vi "Brainstorming Canvas.vi"() -> ()   [LabVIEW 2015]
uses:
  <vilib>/Utility/file.llb/Read Delimited Spreadsheet (I64).vi
  <vilib>/Utility/file.llb/Write Delimited Spreadsheet (I64).vi
  Endigit Library/Endigit.lvlib
panel:
  in  "Current Color":u32(colorbox)=16711680
  in  "New Idea":bool
  in  "stop":bool
  in  "Idea":u16(ring) items=["asdf", "Buff line", "Concentri City", "Death Star", "ex", "Expand", "Lattice", "Line Dancer", "Pods", "SVoT"]
  in  "Canvas":u32[][](array[colorbox])
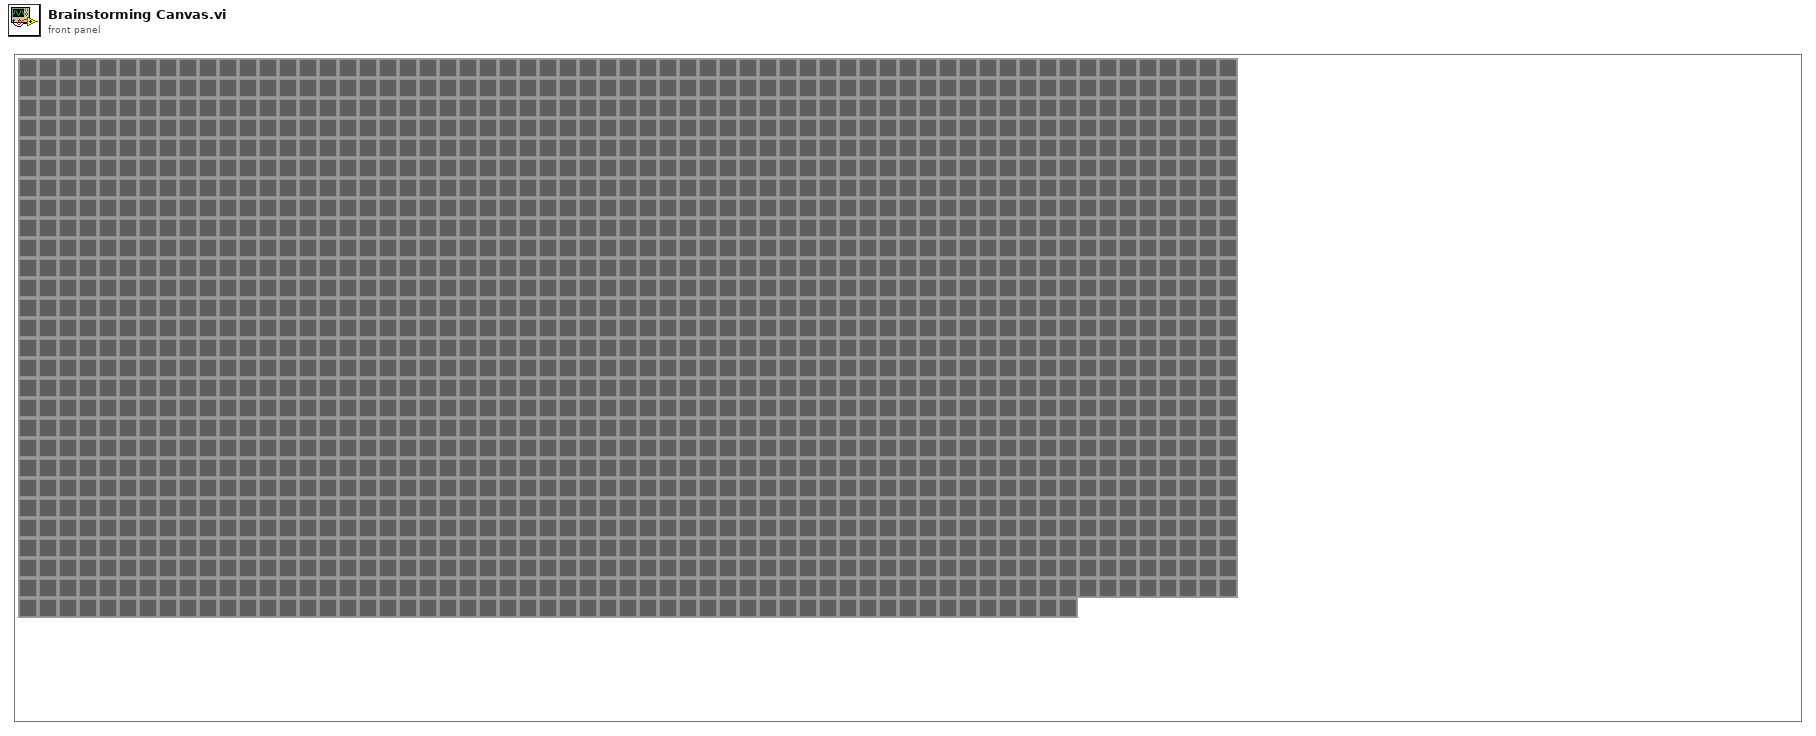
[diagram p1: front panel]
types:
  T1 = typedef "LVPositionTypeDef.ctl" = cluster{"Left":i32, "Top":i32}
  T2 = typedef "LVBoundsTypeDef.ctl" = cluster{"Width":u32, "Height":u32}
  T3 = typedef "LVPoint32TypeDef.ctl" = cluster{"Horizontal":i32, "Vertical":i32}
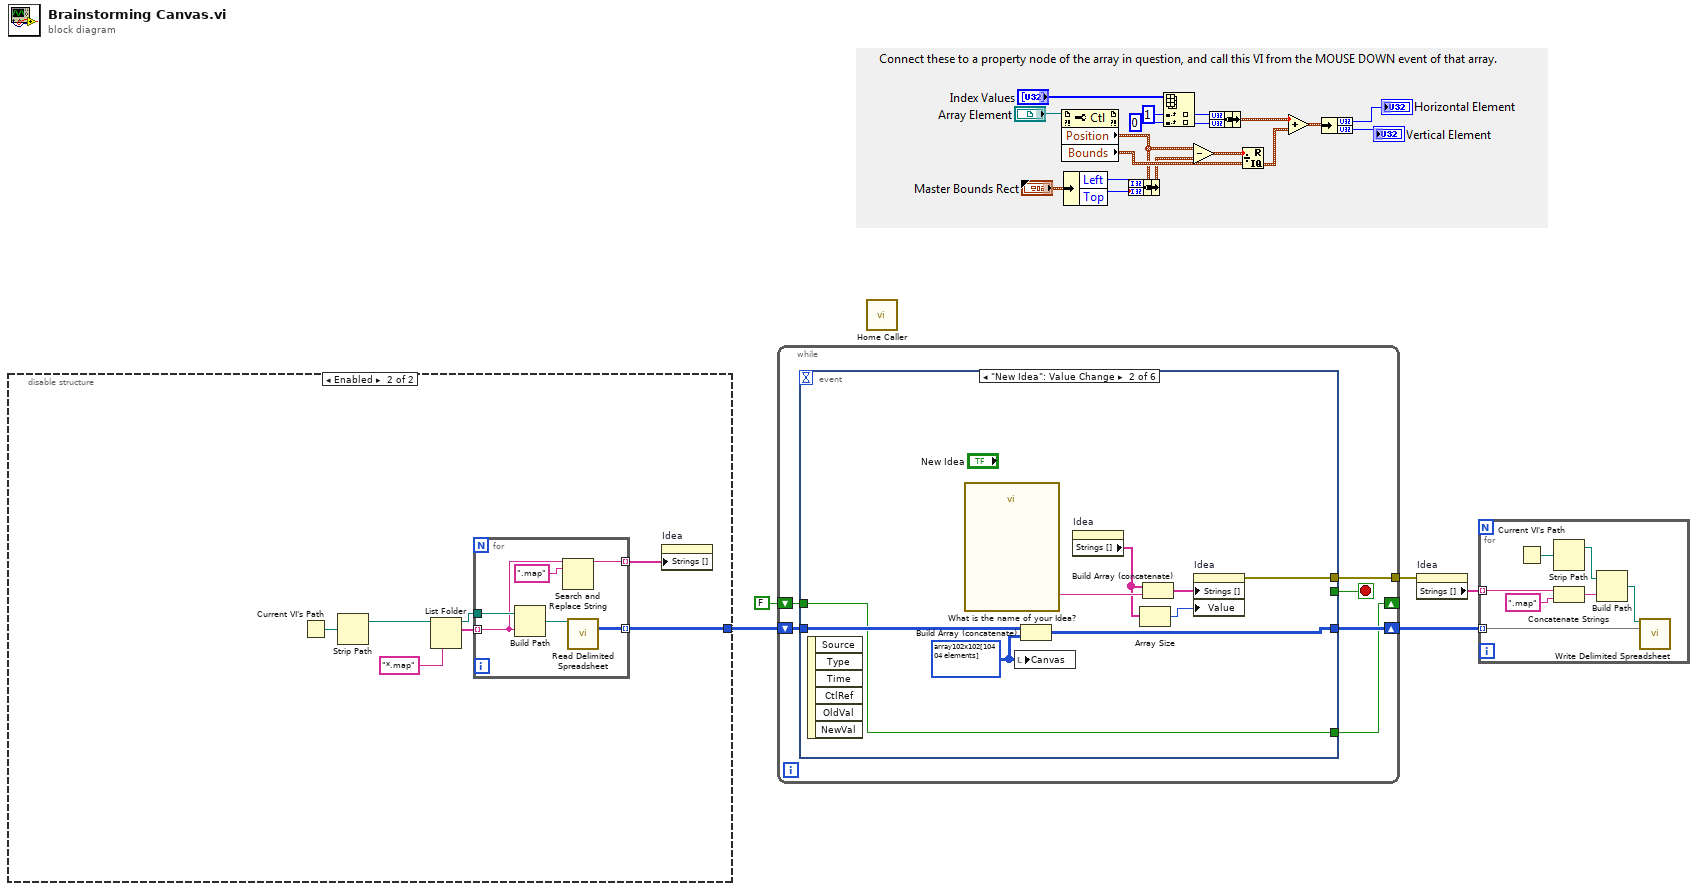
[diagram p0: block diagram]
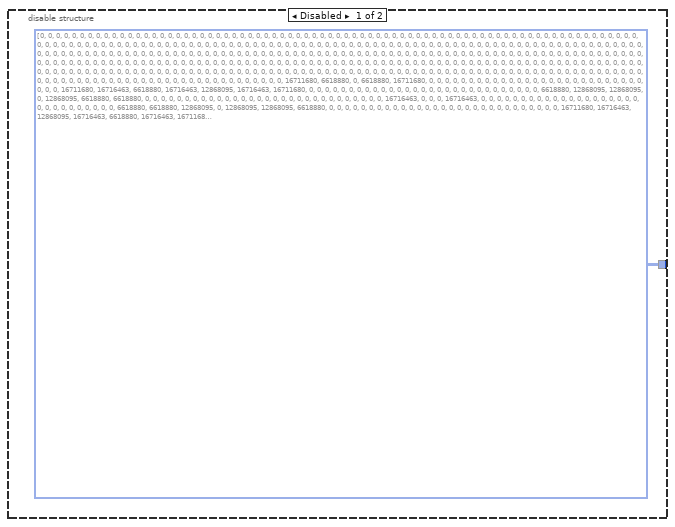
[diagram p2: hidden frame]
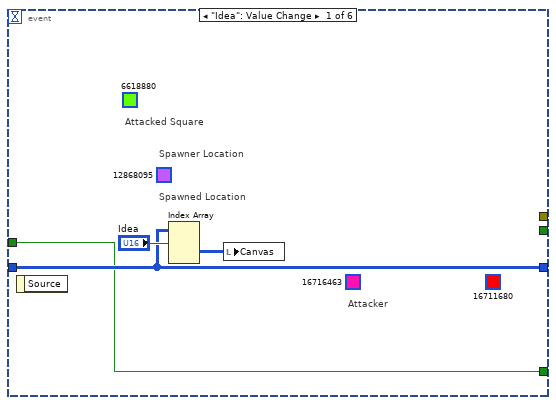
[diagram p3: hidden frame]
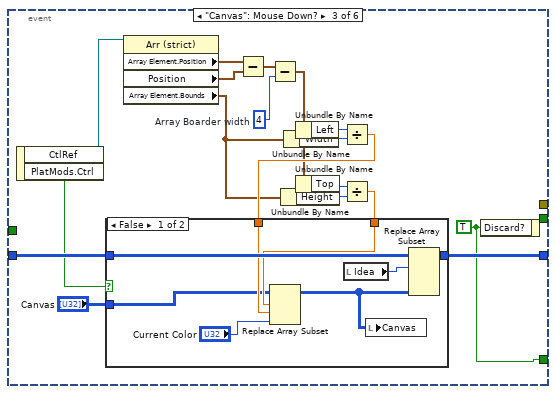
[diagram p4: hidden frame]
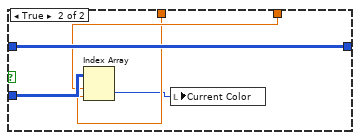
[diagram p5: hidden frame]
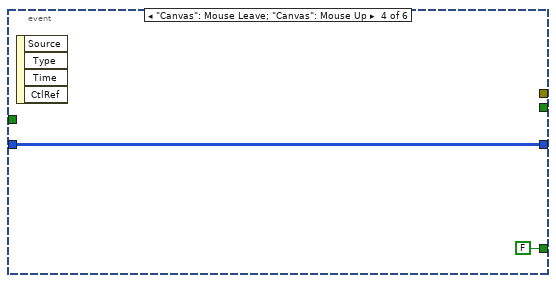
[diagram p6: hidden frame]
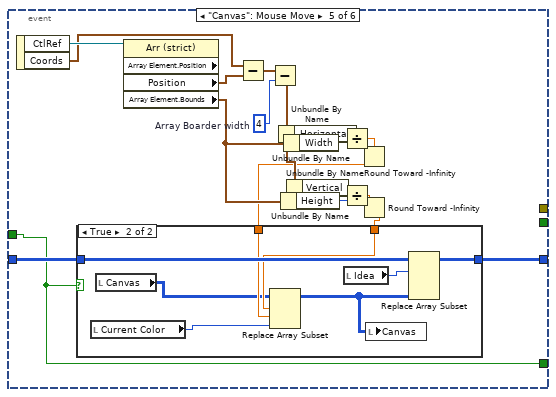
[diagram p7: hidden frame]
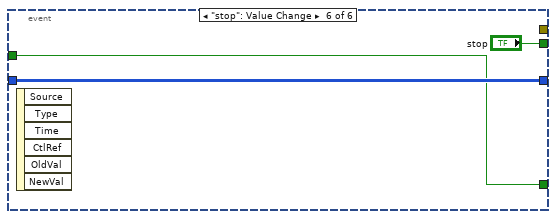
[diagram p9: hidden frame]
diagram:
  n1 = disable-structure shown="Enabled" {
    disable-tunnel: [u32[][][] [[[0, 0, 0, 0, 0, 0, 0, 0, 0, 0, 0, 0, 0, 0, 0, 0, 0, 0, 0, 0, 0, 0, 0, 0, 0, 0, 0, 0, 0, 0, 0, 0, 0, 0, 0, 0], [0, 0, 0, 0, 0, 0, 0, 0, 0, 0, 0, 0, 0, 0, 0, 0, 0, 0, 0, 0, 0, 0, 0, 0, 0, 0, 0, 0, 0, 0, 0, 0, 0, 0, 0, 0], [0, 0, 0, 0, 0, 0, 0, 0, 0, 0, 0, 0, 0, 0, 0, 0, 0, 0, 0, 0, 0, 0, 0, 0, 0, 0, 0, 0, 0, 0, 0, 0, 0, 0, 0, 0], [0, 0, 0, 0, 0, 0, 0, 0, 0, 0, 0, 0, 0, 0, 0, 0, 0, 0, 0, 0, 0, 0, 0, 0, 0, 0, 0, 0, 0, 0, 0, 0, 0, 0, 0, 0], [0, 0, 0, 0, 0, 0, 0, 0, 0, 0, 0, 0, 0, 0, 0, 0, 0, 0, 0, 0, 0, 0, 0, 0, 0, 0, 0, 0, 0, 0, 0, 0, 0, 0, 0, 0], [0, 0, 0, 0, 0, 0, 0, 0, 0, 0, 0, 0, 0, 0, 0, 0, 0, 0, 0, 0, 0, 0, 0, 0, 0, 0, 0, 0, 0, 0, 0, 0, 0, 0, 0, 0], [0, 0, 0, 0, 0, 0, 0, 0, 0, 0, 0, 0, 0, 0, 0, 0, 0, 0, 0, 0, 0, 0, 0, 0, 0, 0, 0, 0, 0, 0, 0, 0, 0, 0, 0, 0], [0, 0, 0, 0, 0, 0, 0, 0, 0, 0, 0, 0, 0, 0, 0, 0, 0, 0, 0, 0, 0, 0, 0, 0, 0, 0, 0, 0, 0, 0, 0, 0, 0, 0, 0, 0], [0, 0, 0, 0, 0, 0, 0, 0, 0, 0, 0, 0, 0, 0, 0, 0, 0, 0, 0, 0, 0, 0, 0, 0, 0, 0, 0, 0, 0, 0, 0, 0, 0, 0, 0, 0], [0, 0, 0, 0, 0, 0, 0, 0, 0, 0, 0, 0, 0, 0, 0, 0, 0, 0, 0, 0, 0, 0, 0, 0, 0, 0, 0, 0, 0, 0, 0, 0, 0, 0, 0, 0], [0, 0, 0, 0, 0, 0, 0, 0, 0, 0, 0, 0, 0, 0, 0, 0, 0, 0, 0, 0, 0, 0, 0, 0, 0, 0, 0, 0, 0, 0, 0, 0, 0, 0, 0, 0], [0, 0, 0, 0, 0, 0, 0, 0, 0, 0, 0, 0, 0, 0, 16711680, 6618880, 0, 6618880, 16711680, 0, 0, 0, 0, 0, 0, 0, 0, 0, 0, 0, 0, 0, 0, 0, 0, 0], [0, 0, 0, 0, 0, 0, 0, 0, 0, 0, 0, 0, 0, 16711680, 16716463, 6618880, 16716463, 12868095, 16716463, 16711680, 0, 0, 0, 0, 0, 0, 0, 0, 0, 0, 0, 0, 0, 0, 0, 0], [0, 0, 0, 0, 0, 0, 0, 0, 0, 0, 0, 0, 0, 6618880, 12868095, 12868095, 0, 12868095, 6618880, 6618880, 0, 0, 0, 0, 0, 0, 0, 0, 0, 0, 0, 0, 0, 0, 0, 0], [0, 0, 0, 0, 0, 0, 0, 0, 0, 0, 0, 0, 0, 0, 16716463, 0, 0, 0, 16716463, 0, 0, 0, 0, 0, 0, 0, 0, 0, 0, 0, 0, 0, 0, 0, 0, 0], [0, 0, 0, 0, 0, 0, 0, 0, 0, 0, 0, 0, 0, 6618880, 6618880, 12868095, 0, 12868095, 12868095, 6618880, 0, 0, 0, 0, 0, 0, 0, 0, 0, 0, 0, 0, 0, 0, 0, 0], [0, 0, 0, 0, 0, 0, 0, 0, 0, 0, 0, 0, 0, 16711680, 16716463, 12868095, 16716463, 6618880, 16716463, 16711680, 0, 0, 0, 0, 0, 0, 0, 0, 0, 0, 0, 0, 0, 0, 0, 0], [0, 0, 0, 0, 0, 0, 0, 0, 0, 0, 0, 0, 0, 0, 16711680, 6618880, 0, 6618880, 16711680, 0, 0, 0, 0, 0, 0, 0, 0, 0, 0, 0, 0, 0, 0, 0, 0, 0], [0, 0, 0, 0, 0, 0, 0, 0, 0, 0, 0, 0, 0, 0, 0, 0, 0, 0, 0, 0, 0, 0, 0, 0, 0, 0, 0, 0, 0, 0, 0, 0, 0, 0, 0, 0], [0, 0, 0, 0, 0, 0, 0, 0, 0, 0, 0, 0, 0, 0, 0, 0, 0, 0, 0, 0, 0, 0, 0, 0, 0, 0, 0, 0, 0, 0, 0, 0, 0, 0, 0, 0], [0, 0, 0, 0, 0, 0, 0, 0, 0, 0, 0, 0, 0, 0, 0, 0, 0, 0, 0, 0, 0, 0, 0, 0, 0, 0, 0, 0, 0, 0, 0, 0, 0, 0, 0, 0], [0, 0, 0, 0, 0, 0, 0, 0, 0, 0, 0, 0, 0, 0, 0, 0, 0, 0, 0, 0, 0, 0, 0, 0, 0, 0, 0, 0, 0, 0, 0, 0, 0, 0, 0, 0], [0, 0, 0, 0, 0, 0, 0, 0, 0, 0, 0, 0, 0, 0, 0, 0, 0, 0, 0, 0, 0, 0, 0, 0, 0, 0, 0, 0, 0, 0, 0, 0, 0, 0, 0, 0], [0, 0, 0, 0, 0, 0, 0, 0, 0, 0, 0, 0, 0, 0, 0, 0, 0, 0, 0, 0, 0, 0, 0, 0, 0, 0, 0, 0, 0, 0, 0, 0, 0, 0, 0, 0], [0, 0, 0, 0, 0, 0, 0, 0, 0, 0, 0, 0, 0, 0, 0, 0, 0, 0, 0, 0, 0, 0, 0, 0, 0, 0, 0, 0, 0, 0, 0, 0, 0, 0, 0, 0], [0, 0, 0, 0, 0, 0, 0, 0, 0, 0, 0, 0, 0, 0, 0, 0, 0, 0, 0, 0, 0, 0, 0, 0, 0, 0, 0, 0, 0, 0, 0, 0, 0, 0, 0, 0], [0, 0, 0, 0, 0, 0, 0, 0, 0, 0, 0, 0, 0, 0, 0, 0, 0, 0, 0, 0, 0, 0, 0, 0, 0, 0, 0, 0, 0, 0, 0, 0, 0, 0, 0, 0], [0, 0, 0, 0, 0, 0, 0, 0, 0, 0, 0, 0, 0, 0, 0, 0, 0, 0, 0, 0, 0, 0, 0, 0, 0, 0, 0, 0, 0, 0, 0, 0, 0, 0, 0, 0], [0, 0, 0, 0, 0, 0, 0, 0, 0, 0, 0, 0, 0, 0, 0, 0, 0, 0, 0, 0, 0, 0, 0, 0, 0, 0, 0, 0, 0, 0, 0, 0, 0, 0, 0, 0]], [[0, 0, 0, 0, 0, 0, 0, 0, 0, 0, 0, 0, 0, 0, 0, 0, 0, 0, 0, 0, 0, 0, 0, 0, 0, 0, 0, 0, 0, 0, 0, 0, 0, 0, 0, 0], [0, 0, 0, 0, 0, 0, 0, 0, 0, 0, 0, 0, 0, 0, 0, 0, 0, 0, 0, 0, 0, 0, 0, 0, 0, 0, 0, 0, 0, 0, 0, 0, 0, 0, 0, 0], [0, 0, 0, 0, 0, 0, 0, 0, 0, 0, 0, 0, 0, 0, 0, 0, 0, 0, 0, 0, 0, 0, 0, 0, 0, 0, 0, 0, 0, 0, 0, 0, 0, 0, 0, 0], [0, 0, 0, 0, 0, 0, 0, 0, 0, 0, 0, 0, 0, 0, 0, 0, 0, 0, 0, 0, 0, 0, 0, 0, 0, 0, 0, 0, 0, 0, 0, 0, 0, 0, 0, 0], [0, 0, 0, 0, 0, 0, 0, 0, 0, 0, 0, 0, 0, 0, 0, 0, 0, 0, 0, 0, 0, 0, 0, 0, 0, 0, 0, 0, 0, 0, 0, 0, 0, 0, 0, 0], [0, 0, 0, 0, 0, 0, 0, 0, 0, 0, 0, 0, 0, 0, 0, 0, 0, 0, 0, 0, 0, 0, 0, 0, 0, 0, 0, 0, 0, 0, 0, 0, 0, 0, 0, 0], [0, 0, 0, 0, 0, 0, 0, 0, 0, 0, 0, 0, 0, 0, 0, 0, 0, 0, 0, 0, 0, 0, 0, 0, 0, 0, 0, 0, 0, 0, 0, 0, 0, 0, 0, 0], [0, 0, 0, 0, 16711680, 16711680, 16711680, 16711680, 16711680, 16711680, 16711680, 16711680, 16711680, 16711680, 0, 0, 0, 0, 0, 0, 0, 0, 0, 0, 0, 0, 0, 0, 0, 0, 0, 0, 0, 0, 0, 0], [0, 0, 16716463, 12868095, 6618880, 6618880, 6618880, 6618880, 6618880, 6618880, 6618880, 6618880, 6618880, 6618880, 12868095, 16716463, 0, 0, 0, 0, 0, 0, 0, 0, 0, 0, 0, 0, 0, 0, 0, 0, 0, 0, 0, 0], [0, 0, 16716463, 12868095, 6618880, 6618880, 6618880, 6618880, 6618880, 6618880, 6618880, 6618880, 6618880, 6618880, 12868095, 16716463, 0, 0, 0, 0, 0, 0, 0, 0, 0, 0, 0, 0, 0, 0, 0, 0, 0, 0, 0, 0], [0, 0, 0, 0, 16711680, 16711680, 16711680, 16711680, 16711680, 16711680, 16711680, 16711680, 16711680, 16711680, 0, 0, 0, 0, 0, 0, 0, 0, 0, 0, 0, 0, 0, 0, 0, 0, 0, 0, 0, 0, 0, 0], [0, 0, 0, 0, 0, 0, 0, 0, 0, 0, 0, 0, 0, 0, 0, 0, 0, 0, 0, 0, 0, 0, 0, 0, 0, 0, 0, 0, 0, 0, 0, 0, 0, 0, 0, 0], [0, 0, 0, 0, 0, 0, 0, 0, 0, 0, 0, 0, 0, 0, 0, 0, 0, 0, 0, 0, 0, 0, 0, 0, 0, 0, 0, 0, 0, 0, 0, 0, 0, 0, 0, 0], [0, 0, 0, 0, 0, 0, 0, 0, 0, 0, 0, 0, 0, 0, 0, 0, 0, 0, 0, 0, 0, 0, 0, 0, 0, 0, 0, 0, 0, 0, 0, 0, 0, 0, 0, 0], [0, 0, 0, 0, 0, 0, 0, 0, 0, 0, 0, 0, 0, 0, 0, 0, 0, 0, 0, 0, 0, 0, 0, 0, 0, 0, 0, 0, 0, 0, 0, 0, 0, 0, 0, 0], [0, 0, 0, 0, 0, 0, 0, 0, 0, 0, 0, 0, 0, 0, 0, 0, 0, 0, 0, 0, 0, 0, 0, 0, 0, 0, 0, 0, 0, 0, 0, 0, 0, 0, 0, 0], [0, 0, 0, 0, 0, 0, 0, 0, 0, 0, 0, 0, 0, 0, 0, 0, 0, 0, 0, 0, 0, 0, 0, 0, 0, 0, 0, 0, 0, 0, 0, 0, 0, 0, 0, 0], [0, 0, 0, 0, 0, 0, 0, 0, 0, 0, 0, 0, 0, 0, 0, 0, 0, 0, 0, 0, 0, 0, 0, 0, 0, 0, 0, 0, 0, 0, 0, 0, 0, 0, 0, 0], [0, 0, 0, 0, 0, 0, 0, 0, 0, 0, 0, 0, 0, 0, 0, 0, 0, 0, 0, 0, 0, 0, 0, 0, 0, 0, 0, 0, 0, 0, 0, 0, 0, 0, 0, 0], [0, 0, 0, 0, 0, 0, 0, 0, 0, 0, 0, 0, 0, 0, 0, 0, 0, 0, 0, 0, 0, 0, 0, 0, 0, 0, 0, 0, 0, 0, 0, 0, 0, 0, 0, 0], [0, 0, 0, 0, 0, 0, 0, 0, 0, 0, 0, 0, 0, 0, 0, 0, 0, 0, 0, 0, 0, 0, 0, 0, 0, 0, 0, 0, 0, 0, 0, 0, 0, 0, 0, 0], [0, 0, 0, 0, 0, 0, 0, 0, 0, 0, 0, 0, 0, 0, 0, 0, 0, 0, 0, 0, 0, 0, 0, 0, 0, 0, 0, 0, 0, 0, 0, 0, 0, 0, 0, 0], [0, 0, 0, 0, 0, 0, 0, 0, 0, 0, 0, 0, 0, 0, 0, 0, 0, 0, 0, 0, 0, 0, 0, 0, 0, 0, 0, 0, 0, 0, 0, 0, 0, 0, 0, 0], [0, 0, 0, 0, 0, 0, 0, 0, 0, 0, 0, 0, 0, 0, 0, 0, 0, 0, 0, 0, 0, 0, 0, 0, 0, 0, 0, 0, 0, 0, 0, 0, 0, 0, 0, 0], [0, 0, 0, 0, 0, 0, 0, 0, 0, 0, 0, 0, 0, 0, 0, 0, 0, 0, 0, 0, 0, 0, 0, 0, 0, 0, 0, 0, 0, 0, 0, 0, 0, 0, 0, 0], [0, 0, 0, 0, 0, 0, 0, 0, 0, 0, 0, 0, 0, 0, 0, 0, 0, 0, 0, 0, 0, 0, 0, 0, 0, 0, 0, 0, 0, 0, 0, 0, 0, 0, 0, 0], [0, 0, 0, 0, 0, 0, 0, 0, 0, 0, 0, 0, 0, 0, 0, 0, 0, 0, 0, 0, 0, 0, 0, 0, 0, 0, 0, 0, 0, 0, 0, 0, 0, 0, 0, 0], [0, 0, 0, 0, 0, 0, 0, 0, 0, 0, 0, 0, 0, 0, 0, 0, 0, 0, 0, 0, 0, 0, 0, 0, 0, 0, 0, 0, 0, 0, 0, 0, 0, 0, 0, 0], [0, 0, 0, 0, 0, 0, 0, 0, 0, 0, 0, 0, 0, 0, 0, 0, 0, 0, 0, 0, 0, 0, 0, 0, 0, 0, 0, 0, 0, 0, 0, 0, 0, 0, 0, 0]]] ("Death Star") w8] -> w2
    frame Disabled {
    }
    frame Enabled {
      n2 = Current VI's Path() -> (path=w10:path)
      n3 = Strip Path(path=w10) -> (stripped path=w7:path)  [unwired: 1 out]
      n4 = List Folder(path=w7, pattern="*.map") -> (path out=w11:path, filenames=w12:string[])  [unwired: 2 in, 2 out]
      n5 = for {
        tunnel: w11 -> [w19]
        tunnel: w12 -> [w15] mode=indexing
        tunnel: [w17] -> w8 mode=indexing
        tunnel: [w14] -> w13 mode=indexing
        n6 = Build Path(base path=w19, name or relative path=w15) -> (appended path=w18:path)
        n7 = Search and Replace String(input string=w15, search string=".map") -> (result string=w14:string)  [unwired: 6 in, 3 out]
        n8 = call-poly <vilib>:"Read Delimited Spreadsheet.vi"("file path (dialog if empty)"=w18) -> ("all rows"=w17:i64[][])  [unwired: 9 in, 5 out]
      }
      n9 = property on="Idea" class="Ring (strict)"("Strings []"=w13) -> ()  [unwired: 2 in, 2 out]
    }
  }
  n10 = while {
    shift-right: [w23] -> w4
    shift-left: w2 -> [w24]
    tunnel: [w22] -> w5
    shift-right: [w20] -> _
    shift-left: FALSE -> [w21]
    stop <- w25 stop-if-true
    n11 = event shown="[1] \"New Idea\": Value Change" {
      selector: _ -> [_ _ _ _ _ _]
      dyn-events: _ -> [_ _ _ _ _ _]
      timeout: _ -> [_ _ _ _ _ _]
      tunnel: [_ _ _ _ _ "stop"] -> w25
      tunnel: w24 -> [w27 w38 w56 w71 w89 w100]
      tunnel: [w27 w35 w55 w71 w88 w100] -> w23
      tunnel: [_ w33 _ _ _ _] -> w22
      tunnel: w21 -> [w26 w32 _ _ w72 w99]
      tunnel: [w26 w32 w39 FALSE ("Discard?") w72 w99] -> w20
      event "Idea": Value Change {
        (unwired) u32 16711680 ("Color Box 17")
        (unwired) u32 6618880 ("Color Box 14")
        (unwired) u32 16716463 ("Color Box 11")
        (unwired) u32 12868095 ("Color Box 12")
        # "Attacked Square"
        # "Attacker"
        # "Spawned Location"
        # "Spawner Location"
        n12 = event-data() -> ()  [unwired: 1 in, 1 out]
        n13 = Index Array(array=w27, index (dim 0)="Idea") -> (element=w28:i64[][])  [unwired: 2 in]
        n14 = local write "Canvas"(w28) -> ()
      }
      event "New Idea": Value Change {
        w34 = u32[][] array102x102[10404 elements] ("Death Star")
        n15 = event-data() -> ()  [unwired: 1 in, 6 out]
        n16 = call "What is the name of your Idea?"() -> ("Idea Name"=w37:string)  [unwired: 17 in, 2 out]
        n17 = local write "Canvas"(w34) -> ()
        n18 = Build Array (concatenate)(w38, w34) -> (w35:i64[][][])
        n19 = property on="Idea" class="Ring (strict)"() -> ("Strings []"=w31:string[])  [unwired: 2 in, 2 out]
        n20 = Array Size(array=w31) -> (size(s)=w30:i32)
        n21 = Build Array (concatenate)(w31, w37) -> (w36:string[])
        n22 = property on="Idea" class="Ring (strict)"("Strings []"=w36, "Value"=w30) -> (error out=w33:errorcluster)  [unwired: 2 in, 1 out]
      }
      event "Canvas": Mouse Down? {
        w51 = 4  # Array Boarder width
        w39 = TRUE ("Discard?")
        n23 = event-data() -> ("CtlRef"=w54:refnum<vi>, "PlatMods.Ctrl"=w41:bool)  [unwired: 1 in]
        n24 = property class="Arr (strict)"(reference=w54) -> ("Array Element.Position"=w42:T1, "Position"=w53:T1, "Array Element.Bounds"=w46:T2)  [unwired: 1 in, 2 out]
        n25 = Subtract(x=w42, y=w53) -> (x-y=w52:T1)
        n26 = Subtract(x=w52, y=w51) -> (x-y=w47:T1)
        n27 = Unbundle By Name(w46) -> ("Height"=w44:u32)
        n28 = Unbundle By Name(w46) -> ("Width"=w49:u32)
        n29 = Unbundle By Name(w47) -> ("Left"=w50:i32)
        n30 = Unbundle By Name(w47) -> ("Top"=w45:i32)
        n31 = Divide(x=w50, y=w49) -> (x/y=w48:dbl)
        n32 = Divide(x=w45, y=w44) -> (x/y=w43:dbl)
        n33 = case shown="False" w41 {
          tunnel: w56 -> [w64 w69]
          tunnel: [w63 w69] -> w55
          tunnel: w48 -> [w60 w66]
          tunnel: w43 -> [w59 w67]
          tunnel: "Canvas" -> [w57 w68]
          frame False {
            n34 = Replace Array Subset(array=w57, new element="Current Color", index (row)=w59, index (col)=w60) -> (w58:u32[][])
            n35 = local read "Idea"() -> (w62:u16)
            n36 = local write "Canvas"(w58) -> ()
            n37 = Replace Array Subset(array=w64, new element=w58, index (dim 0)=w62) -> (w63:i64[][][])  [unwired: 2 in]
          }
          frame True {
            n38 = Index Array(array=w68, index (row)=w67, index (col)=w66) -> (element=w65:u32)
            n39 = local write "Current Color"(w65) -> ()
          }
        }
        n40 = event-data("Discard?"=w39) -> ()  [unwired: 1 in, 1 out]
      }
      event "Canvas": Mouse Leave; "Canvas": Mouse Up {
        n41 = event-data() -> ()  [unwired: 1 in, 4 out]
      }
      event "Canvas": Mouse Move {
        w85 = 4  # Array Boarder width
        n42 = event-data() -> ("CtlRef"=w87:refnum<vi>, "Coords"=w75:T3)  [unwired: 1 in]
        n43 = property class="Arr (strict)" props=["Array Element", "Position", "Position", "Array Element", "Bounds"](reference=w87) -> ("Position"=w76:T1, "Array Element.Bounds"=w80:T2)  [unwired: 1 in, 3 out]
        n44 = Subtract(x=w75, y=w76) -> (x-y=w86:T3)
        n45 = Subtract(x=w86, y=w85) -> (x-y=w81:T3)
        n46 = Unbundle By Name(w81) -> ("Horizontal"=w84:i32)
        n47 = Unbundle By Name(w80) -> ("Height"=w78:u32)
        n48 = Unbundle By Name(w80) -> ("Width"=w83:u32)
        n49 = Unbundle By Name(w81) -> ("Vertical"=w79:i32)
        n50 = Divide(x=w84, y=w83) -> (x/y=w82:dbl)
        n51 = Divide(x=w79, y=w78) -> (x/y=w77:dbl)
        n52 = Round Toward -Infinity(1:w82) -> (0:w73:dbl)
        n53 = Round Toward -Infinity(1:w77) -> (0:w74:dbl)
        n54 = case shown="True" w72 {
          tunnel: w89 -> [w90 w98]
          tunnel: [w90 w97] -> w88
          tunnel: w73 -> [_ w96]
          tunnel: w74 -> [_ w95]
          frame False {
          }
          frame True {
            n55 = local read "Current Color"() -> (w91:u32)
            n56 = local read "Canvas"() -> (w92:u32[][])
            n57 = Replace Array Subset(array=w92, new element=w91, index (row)=w95, index (col)=w96) -> (w93:u32[][])
            n58 = local read "Idea"() -> (w94:u16)
            n59 = local write "Canvas"(w93) -> ()
            n60 = Replace Array Subset(array=w98, new element=w93, index (dim 0)=w94) -> (w97:i64[][][])  [unwired: 2 in]
          }
        }
      }
      event "stop": Value Change {
        n61 = event-data() -> ()  [unwired: 1 in, 6 out]
      }
    }
  }
  n62 = call "Home Caller.vi"() -> ()  [unwired: 11 in]
  n63 = property on="Idea" class="Ring (strict)"(error in=w5) -> ("Strings []"=w3:string[])  [unwired: 1 in, 2 out]
  n64 = for {
    tunnel: w4 -> [w108] mode=indexing
    tunnel: w3 -> [w107] mode=indexing
    n65 = Current VI's Path() -> (path=w103:path)
    n66 = Strip Path(path=w103) -> (stripped path=w102:path)  [unwired: 1 out]
    n67 = Concatenate Strings(w107, ".map" ("string")) -> (w106:string)
    n68 = Build Path(base path=w102, name or relative path=w106) -> (appended path=w104:path)
    n69 = call-poly <vilib>:"Write Delimited Spreadsheet.vi"("file path (dialog if empty)"=w104, "2D data"=w108) -> ()  [unwired: 12 in, 2 out]
  }
